vi "add_experiment_group.vi"(2 "error in (no error)":errorcluster, 3 "Experiment.lvclass":refnum<class "Experiment.lvclass">, 4 "Experiments_group.lvclass in":refnum<class "Experiments_group.lvclass">) -> (0 "error out":errorcluster, 1 "Experiments_group.lvclass out":refnum<class "Experiments_group.lvclass">)   [LabVIEW 2015, in "Experiments_group.lvclass"]
uses:
  Experiments_group.lvclass
  Experiment.lvclass
  Experiments_group.lvclass/Experiments_group.ctl
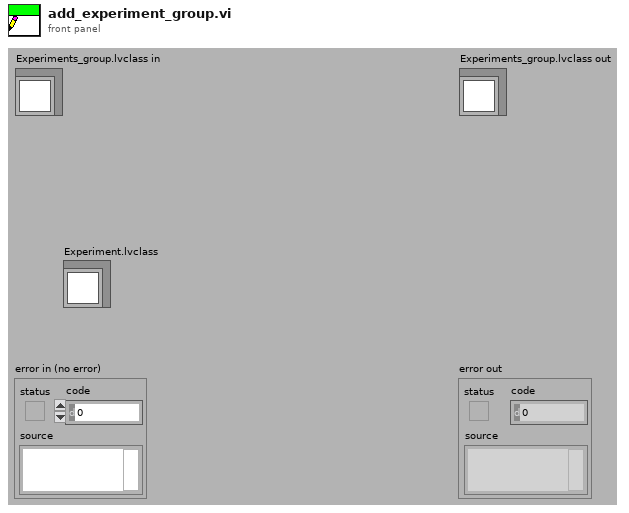
[diagram p1: front panel]
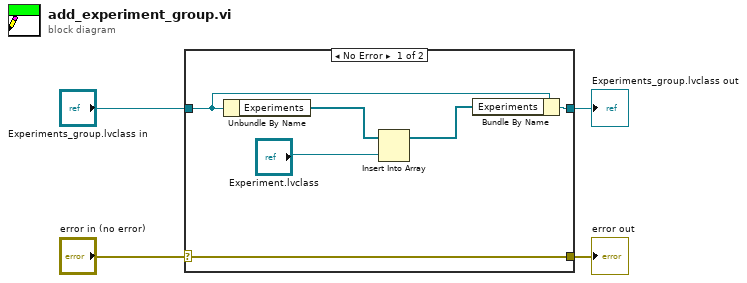
[diagram p0: block diagram]
diagram:
  n1 = case shown="No Error" "error in (no error)" {
    selector: "error in (no error)" -> [w10 w11]
    tunnel: [w10 w11] -> w3
    tunnel: [w9 w12] -> w1
    tunnel: "Experiments_group.lvclass in" -> [w5 w12]
    frame No Error {
      n2 = Unbundle By Name(w5) -> ("Experiments"=w6:refnum<class "Experiment.lvclass">[])
      n3 = Insert Into Array(array=w6, new element="Experiment.lvclass") -> (w7:refnum<class "Experiment.lvclass">[])  [unwired: 1 in]
      n4 = Bundle By Name(cluster=w5, "Experiments"=w7) -> (w9:refnum<class "Experiments_group.lvclass">)
    }
    frame Error {
    }
  }
  "error out" <- w3
  "Experiments_group.lvclass out" <- w1
